vi "Mean_fr_NaN_data for any fraction.vi"(1 "Data":dbl[](array[numeric]) format="%.2f") -> (0 "Mean value":dbl format="%.2f")   [LabVIEW 2022 SP3]
uses:
  <vilib>/Analysis/baseanly.llb/Mean (DBL).vi
  <vilib>/Analysis/NI_AALBase.lvlib
panel:
  # "Removes NaNs from array and computes mean of remaining samples regardless how few samples remain"
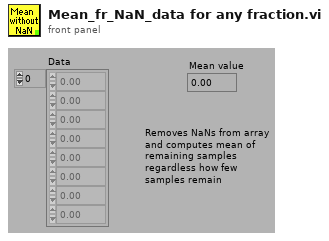
[diagram p1: front panel]
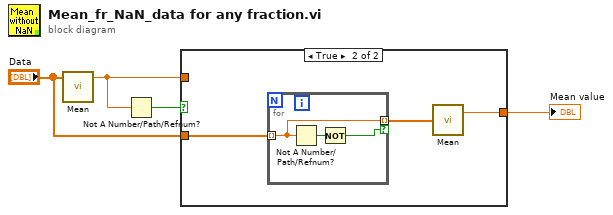
[diagram p0: block diagram]
diagram:
  n1 = call-poly <vilib>:"Mean.vi"("X"="Data") -> ("mean"=w2:dbl)  [unwired: 1 out]
  n2 = Not A Number/Path/Refnum?(number/path/refnum=w2) -> (NaN/Path/Refnum?=w1:bool)
  n3 = case shown="True" w1 {
    tunnel: "Data" -> [_ w8]
    tunnel: [w5 w6] -> w3
    tunnel: w2 -> [w5 _]
    frame False {
    }
    frame True {
      n4 = for {
        tunnel: w8 -> [w10] mode=indexing
        tunnel: [w10] -> w7 mode=indexing if=w9
        n5 = Not A Number/Path/Refnum?(number/path/refnum=w10) -> (NaN/Path/Refnum?=w11:bool)
        n6 = Not(x=w11) -> (.not. x?=w9:bool)
      }
      n7 = call-poly <vilib>:"Mean.vi"("X"=w7) -> ("mean"=w6:dbl)  [unwired: 1 out]
    }
  }
  "Mean value" <- w3
